vi "Solenoids.vi"() -> ()   [LabVIEW 2018]
panel:
  in  "ElevatorSwitch":bool
  in  "BracoSwitch":bool
  in  "CargoSwitch":bool
  in  "HatchSwitch":bool
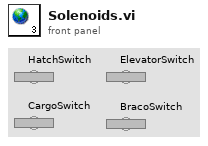
[diagram p1: front panel]
diagram:
